vi "ALTS-2015 File and folder info.vi"(8 "error in (no error)":errorcluster) -> (0 "error out":errorcluster, 1 "DAQ Engine Parameters.ini":path, 2 "INI file path":path, 3 "Report path":path, 4 "ALTS-2015 DAQ DI DO Test VI Path":path, 5 "ALTS Last Test Results File":path, 6 "Test Type Selection Prototype.vi":path, 7 "Info Folder":path, 11 "User.usr path":path)   [LabVIEW 2013]
doc: "Copyright © 2005, Soliton Technologies.\nAll rights reserved."
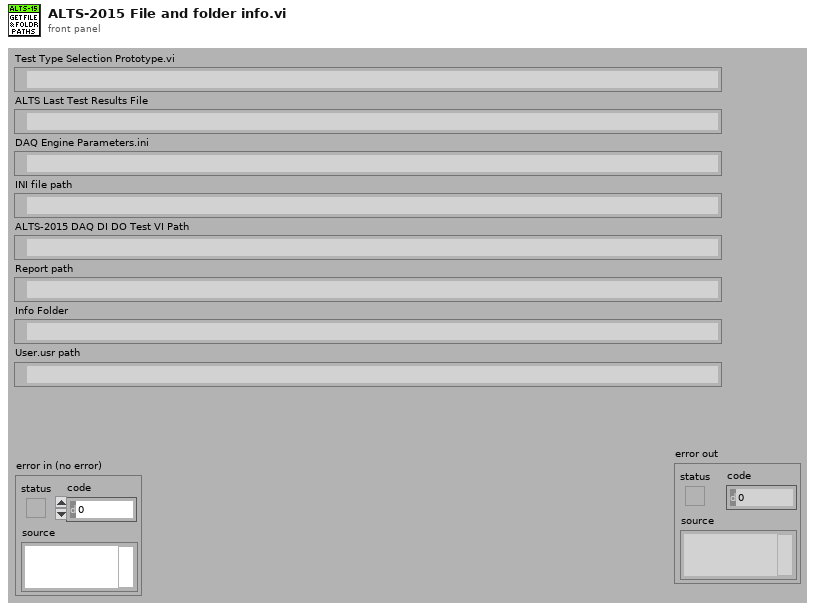
[diagram p1: front panel]
types:
  T1 = enum32{"invalid app kind", "Development System", "Run Time System", "Student Edition", "Embedded LabVIEW", "Evaluation", "Custom"}
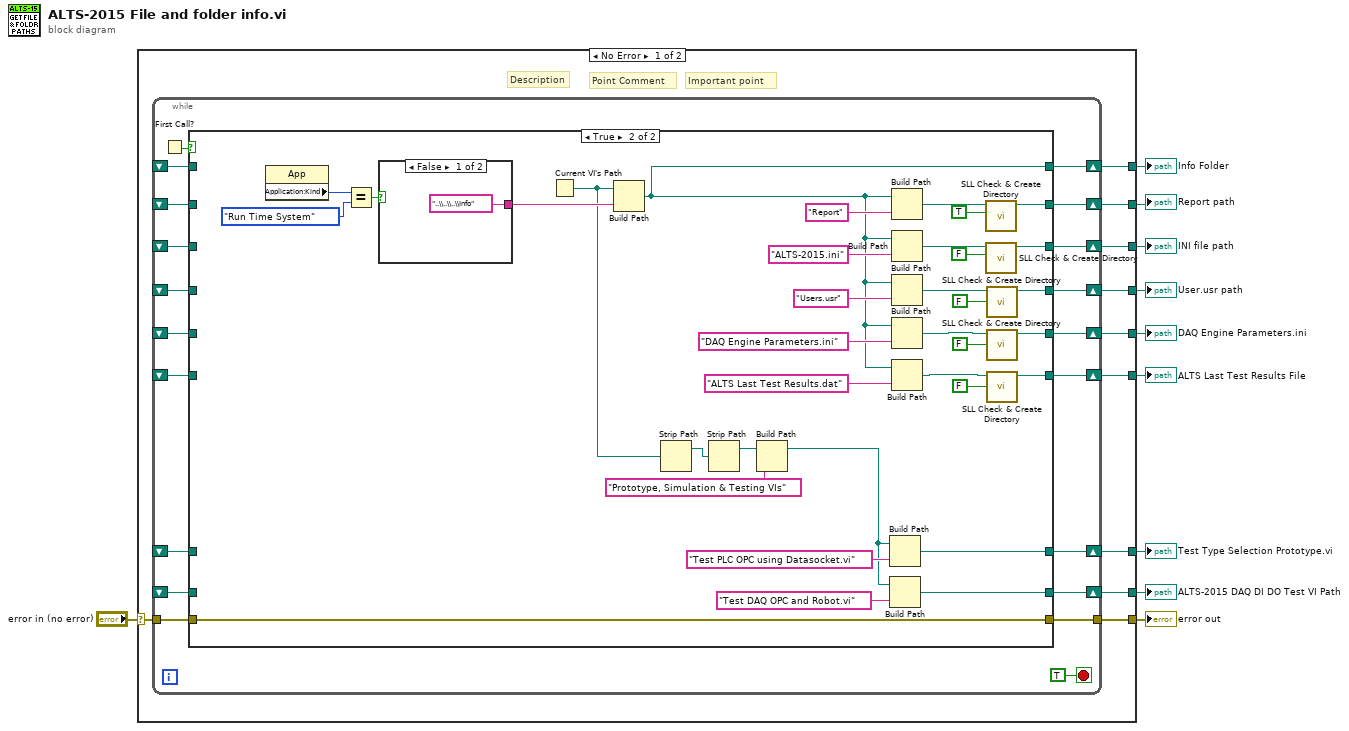
[diagram p0: block diagram]
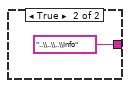
[diagram p3: hidden frame]
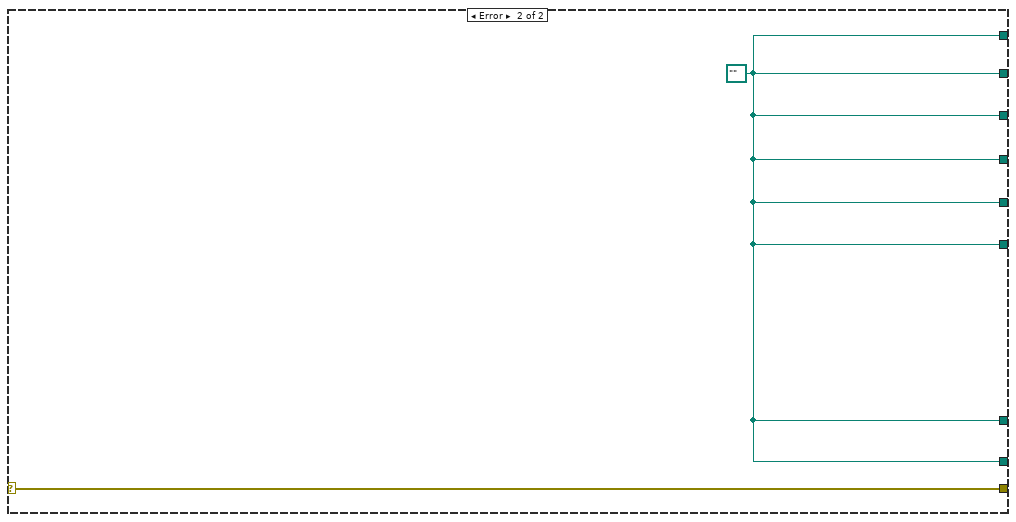
[diagram p4: hidden frame]
diagram:
  n1 = case shown="No Error" "error in (no error)" {
    selector: "error in (no error)" -> [w20 w88]
    tunnel: [w19 w88] -> w9
    tunnel: [w18 w87] -> w8
    tunnel: [w17 w87] -> w7
    tunnel: [w16 w87] -> w6
    tunnel: [w15 w87] -> w5
    tunnel: [w14 w87] -> w4
    tunnel: [w13 w87] -> w3
    tunnel: [w12 w87] -> w2
    tunnel: [w11 w87] -> w1
    frame No Error {
      # "Point Comment"
      # "Important point"
      # "Description"
      n2 = while {
        tunnel: w20 -> [w38]
        tunnel: [w37] -> w19
        shift-right: [w36] -> w18
        shift-left: _ -> [w35]
        shift-right: [w34] -> w17
        shift-left: _ -> [w33]
        shift-right: [w32] -> w16
        shift-left: _ -> [w31]
        shift-right: [w30] -> w15
        shift-left: _ -> [w29]
        shift-right: [w28] -> w14
        shift-left: _ -> [w27]
        shift-right: [w26] -> w13
        shift-left: _ -> [w25]
        shift-right: [w24] -> w12
        shift-left: _ -> [w23]
        shift-right: [w22] -> w11
        shift-left: _ -> [w21]
        stop <- TRUE stop-if-true
        n3 = First Call?() -> (First Call?: T/F=w39:bool)
        n4 = case shown="True" w39 {
          tunnel: w38 -> [w49 w80]
          tunnel: [w49 w80] -> w37
          tunnel: [w48 w76] -> w36
          tunnel: w35 -> [w48 _]
          tunnel: [w47 w74] -> w34
          tunnel: w33 -> [w47 _]
          tunnel: [w46 w55] -> w32
          tunnel: w31 -> [w46 _]
          tunnel: [w45 w68] -> w30
          tunnel: w29 -> [w45 _]
          tunnel: [w44 w65] -> w28
          tunnel: w27 -> [w44 _]
          tunnel: [w43 w61] -> w26
          tunnel: w25 -> [w43 _]
          tunnel: [w42 w57] -> w24
          tunnel: w23 -> [w42 _]
          tunnel: [w41 w52] -> w22
          tunnel: w21 -> [w41 _]
          frame False {
          }
          frame True {
            n5 = property class="App"() -> ("Application:Kind"=w82:T1)  [unwired: 2 in, 2 out]
            n6 = Equal?(x=w82, y=T1."Run Time System") -> (x = y?=w79:bool)
            n7 = case shown="False" w79 {
              tunnel: ["..\\..\\..\\Info" ("name or relative path") "..\\..\\..\\Info" ("name or relative path")] -> w83
              frame False {
              }
              frame True {
              }
            }
            n8 = Current VI's Path() -> (path=w64:path)
            n9 = Build Path(base path=w64, name or relative path=w83) -> (appended path=w55:path)
            n10 = Strip Path(path=w64) -> (stripped path=w63:path)  [unwired: 1 out]
            n11 = Strip Path(path=w63) -> (stripped path=w53:path)  [unwired: 1 out]
            n12 = Build Path(base path=w53, name or relative path="Prototype, Simulation & Testing VIs") -> (appended path=w51:path)
            n13 = Build Path(base path=w51, name or relative path="Test PLC OPC using Datasocket.vi") -> (appended path=w52:path)
            n14 = Build Path(base path=w51, name or relative path="Test DAQ OPC and Robot.vi") -> (appended path=w61:path)
            n15 = Build Path(base path=w55, name or relative path="Report") -> (appended path=w77:path)
            n16 = Build Path(base path=w55, name or relative path="ALTS-2015.ini") -> (appended path=w72:path)
            n17 = Build Path(base path=w55, name or relative path="Users.usr") -> (appended path=w69:path)
            n18 = Build Path(base path=w55, name or relative path="DAQ Engine Parameters.ini") -> (appended path=w59:path)
            n19 = Build Path(base path=w55, name or relative path="ALTS Last Test Results.dat") -> (appended path=w56:path)
            n20 = call <userlib>:"SLL Check & Create Directory.vi"("Path is Directory? (F=No)"=TRUE, "Path"=w77) -> ("Dup Path out"=w76:path)  [unwired: 8 in, 1 out]
            n21 = call <userlib>:"SLL Check & Create Directory.vi"("Path is Directory? (F=No)"=FALSE, "Path"=w72) -> ("Dup Path out"=w74:path)  [unwired: 8 in, 1 out]
            n22 = call <userlib>:"SLL Check & Create Directory.vi"("Path is Directory? (F=No)"=FALSE, "Path"=w69) -> ("Dup Path out"=w68:path)  [unwired: 8 in, 1 out]
            n23 = call <userlib>:"SLL Check & Create Directory.vi"("Path is Directory? (F=No)"=FALSE, "Path"=w59) -> ("Dup Path out"=w65:path)  [unwired: 8 in, 1 out]
            n24 = call <userlib>:"SLL Check & Create Directory.vi"("Path is Directory? (F=No)"=FALSE, "Path"=w56) -> ("Dup Path out"=w57:path)  [unwired: 8 in, 1 out]
          }
        }
      }
    }
    frame Error {
      w87 = path "" ("appended path")
    }
  }
  "error out" <- w9
  "Report path" <- w8
  "INI file path" <- w7
  "Info Folder" <- w6
  "User.usr path" <- w5
  "DAQ Engine Parameters.ini" <- w4
  "ALTS-2015 DAQ DI DO Test VI Path" <- w3
  "ALTS Last Test Results File" <- w2
  "Test Type Selection Prototype.vi" <- w1
